vi "saveDataNodeBegin.vi"(8 "error in (no error)":errorcluster, 9 "indent":i32, 10 "XML Refnum in":refnum<file>, 11 "Parameters in":refnum<class "Parameters.lvclass">) -> (0 "error out":errorcluster, 2 "XML Refnum out":refnum<file>, 3 "Parameters out":refnum<class "Parameters.lvclass">)   [LabVIEW 2013, in "Parameters.lvclass"]
doc: "Begins the process of saving a xceData Node to an XML formatted file."
uses:
  Parameters.lvclass
  xCE/xceNode/xceNode.lvclass
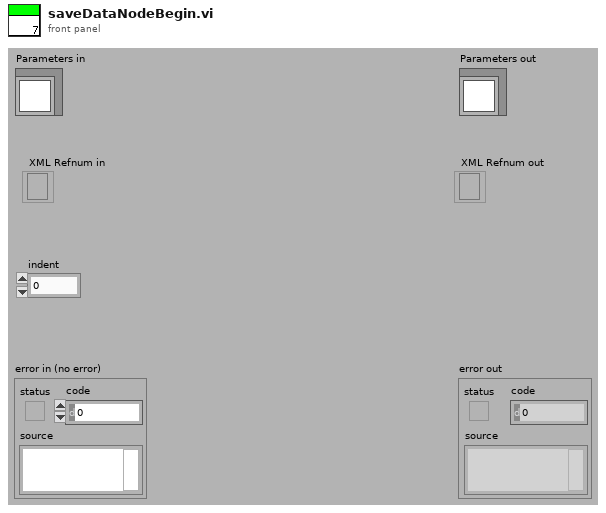
[diagram p1: front panel]
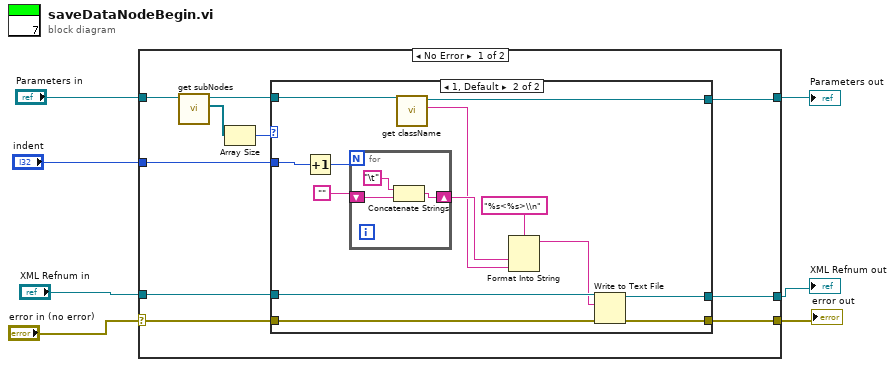
[diagram p0: block diagram]
diagram:
  n1 = case shown="No Error" "error in (no error)" {
    selector: "error in (no error)" -> [w16 w38]
    tunnel: "Parameters in" -> [w11 w39]
    tunnel: "indent" -> [w12 _]
    tunnel: [w17 w39] -> w2
    tunnel: "XML Refnum in" -> [w15 w37]
    tunnel: [w14 w37] -> w3
    tunnel: [w13 w38] -> w4
    frame No Error {
      n2 = call "get subNodes.vi"("xceNode in"=w11) -> ("subNodes[]*"=w9:refnum<data-value>[], "xceNode out"=w10:refnum<class "Parameters.lvclass">)  [unwired: 8 in, 1 out]
      n3 = Array Size(array=w9) -> (size(s)=w8:i32)
      n4 = case shown="1, Default" w8 {
        tunnel: [w20 w29] -> w17
        tunnel: w16 -> [w18 w28]
        tunnel: w15 -> [w19 w27]
        tunnel: [w19 w26] -> w14
        tunnel: [w18 w25] -> w13
        tunnel: w12 -> [_ w23]
        tunnel: w10 -> [w20 w21]
        frame 0 {
          # "No parameters, do not save anything"
        }
        frame 1, Default {
          n5 = Increment(x=w23) -> (x+1=w22:i32)
          n6 = for {
            N: w22 -> [_]
            shift-right: [w36] -> w32
            shift-left: "" -> [w35]
            n7 = Concatenate Strings("\t", w35) -> (w36:string)
          }
          n8 = call "get className.vi"("xceNode in"=w21) -> ("Class name"=w30:string, "xceNode out"=w29:refnum<class "Parameters.lvclass">)  [unwired: 8 in, 1 out]
          n9 = Format Into String(format string="%s<%s>\\n", w32, w30) -> (resulting string=w24:string)  [unwired: 2 in, 1 out]
          n10 = Write to Text File(file (use dialog)=w27, text=w24, error in=w28) -> (refnum out=w26:refnum<file>, error out=w25:errorcluster)  [unwired: 1 in, 1 out]
        }
      }
    }
    frame Error {
    }
  }
  "error out" <- w4
  "Parameters out" <- w2
  "XML Refnum out" <- w3
